vi "Set Mode.vi"(8 "error in (no error)":errorcluster, 9 "LockToLS":T1, 10 "Mode":T2=enum."Run", 11 "FP Controls in":refnum<class "FP Controls.lvclass">) -> (0 "error out":errorcluster, 3 "FP Controls out":refnum<class "FP Controls.lvclass">)   [LabVIEW 2012, in "Configuration Grandmaster.lvlib" / "FP Controls.lvclass"]
uses:
  FP Controls.lvclass
  Common/Controls/DAQMan Mode.ctl
  Common/Controls/LS Lock Sizes.ctl
  FP Controls.lvclass/FP Controls.ctl
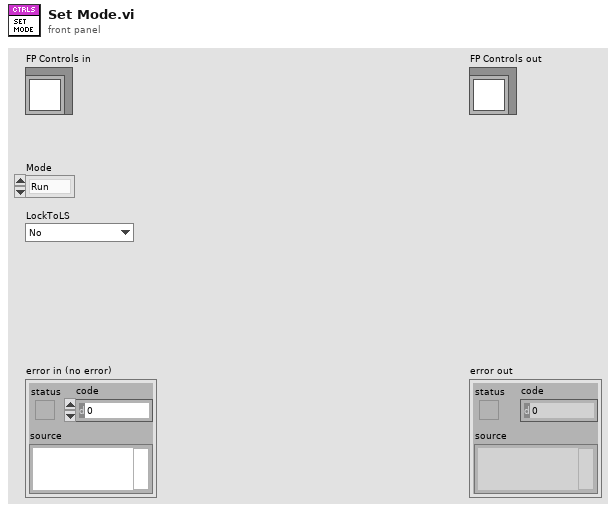
[diagram p1: front panel]
types:
  T1 = typedef "LS Lock Sizes.ctl" = enum16{"No", "250ms", "500ms", "1s"}
  T2 = typedef "DAQMan Mode.ctl" = enum16{"Cfg", "Run", "Shutting Down"}
  T3 = enum8{"Enabled", "Disabled", "Disabled and Grayed Out"}
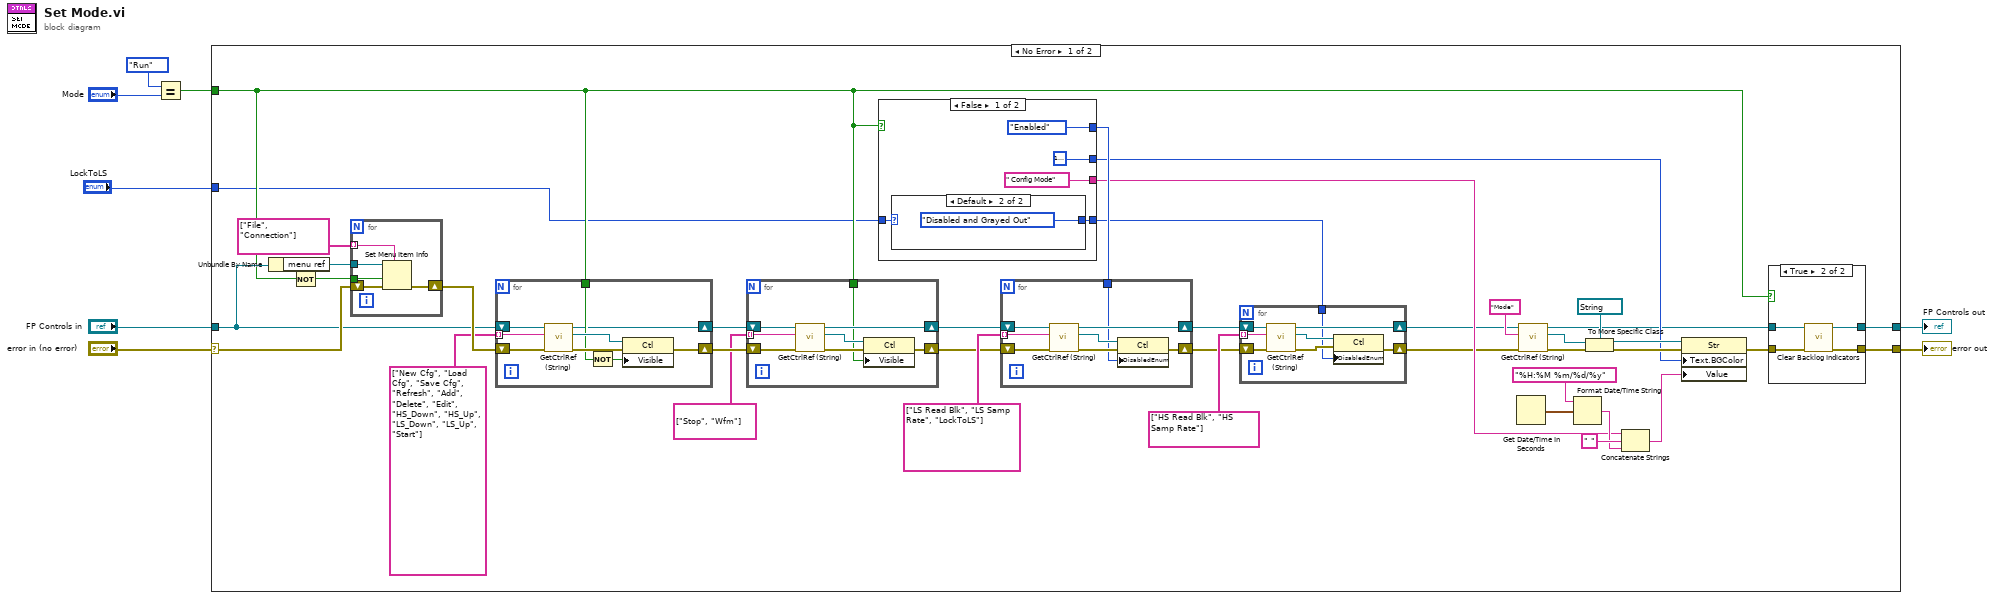
[diagram p0: block diagram]
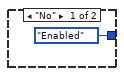
[diagram p3: hidden frame]
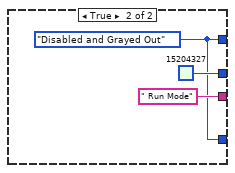
[diagram p4: hidden frame]
diagram:
  n1 = Equal?(x=DAQMan_Mode."Run", y="Mode") -> (x = y?=w3:bool)
  n2 = case shown="No Error" "error in (no error)" {
    selector: "error in (no error)" -> [w22 w103]
    tunnel: [w18 w103] -> w7
    tunnel: [w17 w102] -> w5
    tunnel: "FP Controls in" -> [w21 w102]
    tunnel: w3 -> [w16 _]
    tunnel: "LockToLS" -> [w9 _]
    frame No Error {
      n3 = Unbundle By Name(w21) -> ("menu ref"=w20:refnum<k9>)
      n4 = Not(x=w16) -> (.not. x?=w19:bool)
      n5 = for {
        tunnel: w19 -> [w64]
        tunnel: w20 -> [w63]
        shift-right: [w65] -> w24
        shift-left: w22 -> [w66]
        tunnel: string[] ["File", "Connection"] -> [w62] mode=indexing
        n6 = Set Menu Item Info(7:w62, 8:w66, 9:w64, 11:w63) -> (0:w65:errorcluster)  [unwired: 3 in, 1 out]
      }
      n7 = for {
        shift-right: [w94] -> w44
        shift-left: w24 -> [w100]
        tunnel: string[] ["New Cfg", "Load Cfg", "Save Cfg", "Refresh", "Add", "Delete", "Edit", "HS_Down", "HS_Up", "LS_Down", "LS_Up", "Start"] -> [w99] mode=indexing
        tunnel: w16 -> [w95]
        shift-right: [w93] -> w45
        shift-left: w21 -> [w101]
        n8 = call "GetCtrlRef (String).vi"("error in (no error)"=w100, "FP Control"=w99, "FP Controls in"=w101) -> ("error out"=w98:errorcluster, "Ctrl Ref"=w97:refnum<vi>, "FP Controls out"=w93:refnum<class "FP Controls.lvclass">)  [unwired: 6 in]
        n9 = Not(x=w95) -> (.not. x?=w96:bool)
        n10 = property class="Ctl"(reference=w97, error in=w98, "Visible"=w96) -> (error out=w94:errorcluster)  [unwired: 1 out]
      }
      n11 = for {
        shift-right: [w69] -> w43
        shift-left: w44 -> [w73]
        tunnel: string[] ["Stop", "Wfm"] -> [w72] mode=indexing
        shift-right: [w68] -> w42
        shift-left: w45 -> [w74]
        tunnel: w16 -> [w67]
        n12 = call "GetCtrlRef (String).vi"("error in (no error)"=w73, "FP Control"=w72, "FP Controls in"=w74) -> ("error out"=w71:errorcluster, "Ctrl Ref"=w70:refnum<vi>, "FP Controls out"=w68:refnum<class "FP Controls.lvclass">)  [unwired: 6 in]
        n13 = property class="Ctl"(reference=w70, error in=w71, "Visible"=w67) -> (error out=w69:errorcluster)  [unwired: 1 out]
      }
      n14 = case shown="False" w16 {
        tunnel: [T3."Enabled" ("Disabled") w90] -> w46
        tunnel: [" Config Mode" " Run Mode"] -> w29
        tunnel: [u32 16777225 u32 15204327] -> w34
        tunnel: [w83 w90] -> w10
        tunnel: w9 -> [w84 _]
        frame False {
          n15 = case shown="Default" w84 {
            tunnel: [T3."Enabled" ("Disabled") T3."Disabled and Grayed Out" ("Disabled")] -> w83
            frame "No" {
            }
            frame Default {
            }
          }
        }
        frame True {
          w90 = T3."Disabled and Grayed Out" ("Disabled")
        }
      }
      n16 = for {
        shift-right: [w77] -> w13
        shift-left: w43 -> [w81]
        tunnel: string[] ["LS Read Blk", "LS Samp Rate", "LockToLS"] -> [w80] mode=indexing
        shift-right: [w76] -> w14
        shift-left: w42 -> [w82]
        tunnel: w46 -> [w75]
        n17 = call "GetCtrlRef (String).vi"("error in (no error)"=w81, "FP Control"=w80, "FP Controls in"=w82) -> ("error out"=w79:errorcluster, "Ctrl Ref"=w78:refnum<vi>, "FP Controls out"=w76:refnum<class "FP Controls.lvclass">)  [unwired: 6 in]
        n18 = property class="Ctl"(reference=w78, error in=w79, "DisabledEnum"=w75) -> (error out=w77:errorcluster)  [unwired: 1 out]
      }
      n19 = for {
        tunnel: w10 -> [w50]
        shift-right: [w54] -> w12
        shift-left: w14 -> [w51]
        shift-right: [w55] -> w11
        shift-left: w13 -> [w49]
        tunnel: string[] ["HS Read Blk", "HS Samp Rate"] -> [w48] mode=indexing
        n20 = call "GetCtrlRef (String).vi"("error in (no error)"=w49, "FP Control"=w48, "FP Controls in"=w51) -> ("error out"=w53:errorcluster, "Ctrl Ref"=w52:refnum<vi>, "FP Controls out"=w54:refnum<class "FP Controls.lvclass">)  [unwired: 6 in]
        n21 = property class="Ctl"(reference=w52, error in=w53, "DisabledEnum"=w50) -> (error out=w55:errorcluster)  [unwired: 1 out]
      }
      n22 = Get Date/Time In Seconds() -> (seconds since 1Jan1904=w30:timestamp)
      n23 = call "GetCtrlRef (String).vi"("error in (no error)"=w11, "FP Control"="Mode", "FP Controls in"=w12) -> ("error out"=w36:errorcluster, "Ctrl Ref"=w35:refnum<vi>, "FP Controls out"=w26:refnum<class "FP Controls.lvclass">)  [unwired: 6 in]
      n24 = Format Date/Time String(time format string (%c)="%H:%M %m/%d/%y", seconds (now)=w30) -> (date/time string=w32:string)  [unwired: 1 in]
      n25 = To More Specific Class(target class=refnum<vi> refnum ("Mode"), reference=w35, error in=w36) -> (specific class reference=w38:refnum<vi>, error out=w39:errorcluster)
      n26 = Concatenate Strings(w29, " " ("string"), w32) -> (w28:string)
      n27 = property class="Str"(reference=w38, error in=w39, "Text.BGColor"=w34, "Value"=w28) -> (error out=w27:errorcluster)  [unwired: 1 out]
      n28 = case shown="True" w16 {
        tunnel: w27 -> [w56 w61]
        tunnel: w26 -> [w57 w60]
        tunnel: [w56 w59] -> w18
        tunnel: [w57 w58] -> w17
        frame False {
        }
        frame True {
          n29 = call "Clear Backlog Indicators.vi"("error in (no error)"=w61, "FP Controls in"=w60) -> ("error out"=w59:errorcluster, "FP Controls out"=w58:refnum<class "FP Controls.lvclass">)  [unwired: 8 in]
        }
      }
    }
    frame Error {
    }
  }
  "error out" <- w7
  "FP Controls out" <- w5
